vi "Merge_channel_names.vi"(0 "Preferred Channel array":string[](array[string]), 1 "Channel array":string[](array[string])) -> (2 "Merged Channels":string[](array[string]), 3 "Preferred Channels Changed?":bool, 4 "Channel Array Changed?":bool)   [LabVIEW 2015]
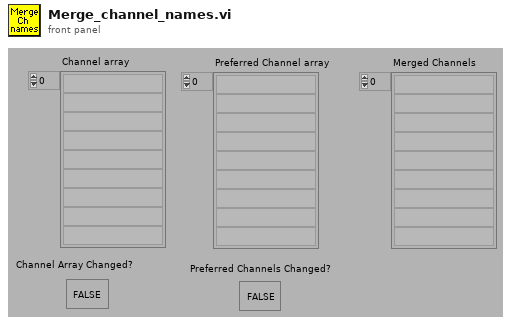
[diagram p1: front panel]
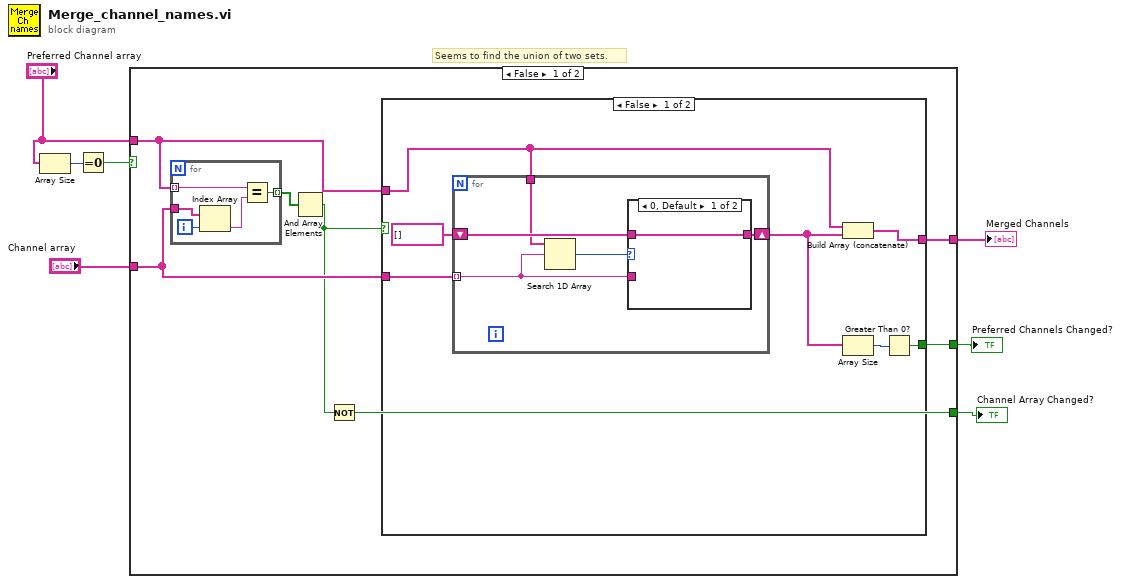
[diagram p0: block diagram]
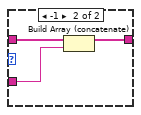
[diagram p2: hidden frame]
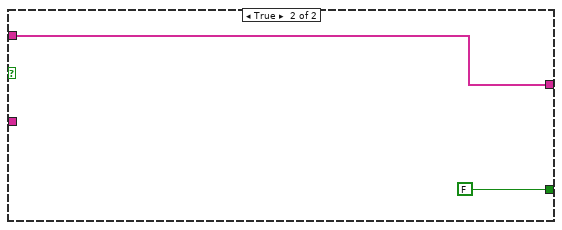
[diagram p3: hidden frame]
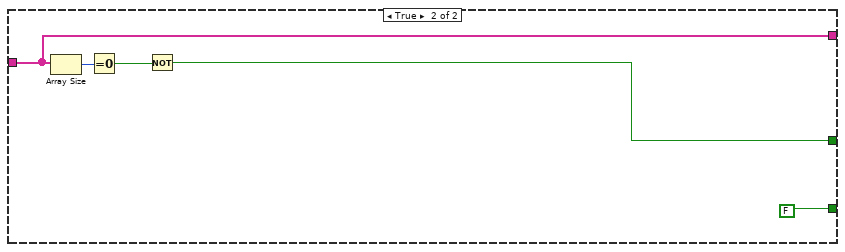
[diagram p4: hidden frame]
diagram:
  # "Seems to find the union of two sets."
  n1 = Array Size(array="Preferred Channel array") -> (size(s)=w4:i32)
  n2 = Equal To 0?(x=w4) -> (x = 0?=w2:bool)
  n3 = case shown="False" w2 {
    tunnel: [w14 w38] -> w7
    tunnel: [w13 w41] -> w6
    tunnel: "Channel array" -> [w12 w41]
    tunnel: [w8 FALSE] -> w1
    tunnel: "Preferred Channel array" -> [w9 _]
    frame False {
      n4 = for {
        tunnel: w9 -> [w19] mode=indexing
        tunnel: w12 -> [w17]
        tunnel: [w15] -> w11 mode=indexing
        i -> [w18]
        n5 = Index Array(array=w17, index=w18) -> (element=w16:string)
        n6 = Equal?(x=w19, y=w16) -> (x = y?=w15:bool)
      }
      n7 = And Array Elements(Boolean array=w11) -> (logical AND=w10:bool)
      n8 = Not(x=w10) -> (.not. x?=w8:bool)
      n9 = case shown="False" w10 {
        tunnel: w12 -> [w26 _]
        tunnel: w9 -> [w25 w37]
        tunnel: [w24 w37] -> w13
        tunnel: [w23 FALSE] -> w14
        frame False {
          n10 = for {
            shift-right: [w29] -> w20
            shift-left: string[] [] -> [w31]
            tunnel: w26 -> [w30] mode=indexing
            tunnel: w25 -> [w28]
            n11 = Search 1D Array(1D array=w28, element=w30) -> (index of element=w27:i32)  [unwired: 1 out]
            n12 = case shown="0, Default" w27 {
              tunnel: w31 -> [w32 w35]
              tunnel: w30 -> [_ w34]
              tunnel: [w32 w33] -> w29
              frame 0, Default {
              }
              frame -1 {
                n13 = Build Array (concatenate)(w35, w34) -> (w33:string[])
              }
            }
          }
          n14 = Build Array (concatenate)(w25, w20) -> (w24:string[])
          n15 = Array Size(array=w20) -> (size(s)=w21:i32)
          n16 = Greater Than 0?(x=w21) -> (x > 0?=w23:bool)
        }
        frame True {
        }
      }
    }
    frame True {
      n17 = Array Size(array=w41) -> (size(s)=w42:i32)
      n18 = Equal To 0?(x=w42) -> (x = 0?=w39:bool)
      n19 = Not(x=w39) -> (.not. x?=w38:bool)
    }
  }
  "Merged Channels" <- w6
  "Preferred Channels Changed?" <- w7
  "Channel Array Changed?" <- w1
